vi "Configure Range.vi"(0 "VISA resource name":refnum<visa-resource-name>, 1 "Unit Address (1)":u8=1 min=1 max=254, 5 "Range High (0)":sgl, 9 "Range Low (0)":sgl, 11 "error in (no error)":errorcluster) -> (4 "VISA resource name out":refnum<visa-resource-name>, 15 "error out":errorcluster)   [LabVIEW 2010, in "Eurotherm 32xx Series.lvlib"]
doc: "This VI sets the limits of input level.\n\nThe range limits are the outer setpoint limits for the load you are controlling, and may be used to set a safe range for operator setpoint adjustment. Range limits are automatically clipped to the range of the sensor you are using. \n\nRange limits are also used in conjunction with the Linear Input High and Low values to set the display range for linear inputs."
uses:
  <instrlib>/Eurotherm 32xx Series/Eurotherm 32xx Series.lvlib
panel:
  # "Range High"
  # "Range Low"
  # "Sensor Input Range"
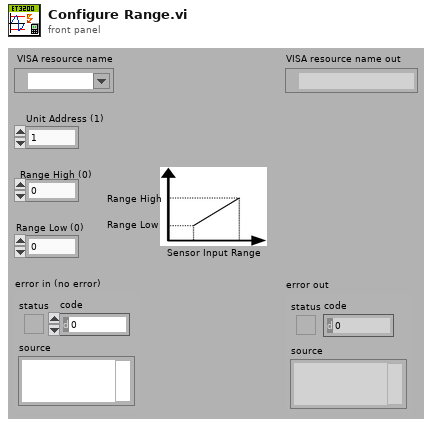
[diagram p1: front panel]
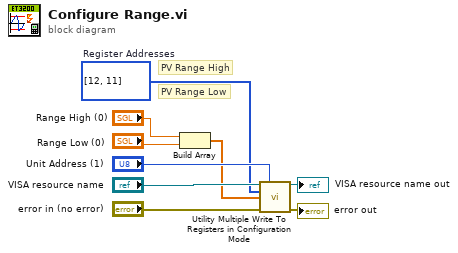
[diagram p0: block diagram]
diagram:
  w3 = u16[] [12, 11]  # Register Addresses
  # "PV Range Low"
  # "PV Range High"
  n1 = Build Array("Range High (0)", "Range Low (0)") -> (w2:sgl[])
  n2 = call <instrlib>:"Utility Multiple Write To Registers in Configuration Mode.vi"("VISA resource name"="VISA resource name", "Unit Address (1)"="Unit Address (1)", "Registers Addresses (0)"=w3, "Data (0)"=w2, "error in (no error)"="error in (no error)") -> ("VISA resource name out"=→"VISA resource name out":refnum<visa-resource-name>, "error out"=→"error out":errorcluster)  [unwired: 9 in]
